vi "TimeStamp To String.vi"(8 "error in (no error)":errorcluster, 11 "Time Stamp":timestamp) -> (0 "error out":errorcluster, 3 "Time string":string)   [LabVIEW 2020, in "Data.lvlib" / "Time Stamp.lvclass"]
doc: "Format a Time Stamp into a String with the format: YYYY-MM-DD hh:mm:ss.ddd"
uses:
  Time Stamp.lvclass
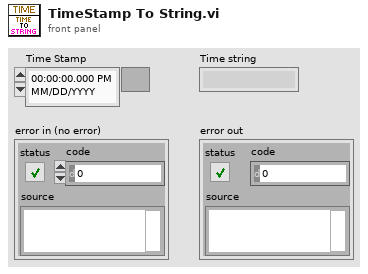
[diagram p1: front panel]
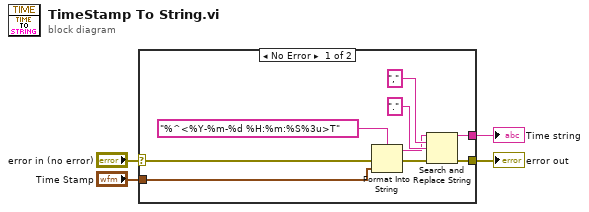
[diagram p0: block diagram]
diagram:
  n1 = case shown="No Error" "error in (no error)" {
    selector: "error in (no error)" -> [w7 w14]
    tunnel: [w13 _] -> w4
    tunnel: [w12 w14] -> w3
    tunnel: "Time Stamp" -> [w5 _]
    frame No Error {
      n2 = Format Into String(format string="%^<%Y-%m-%d %H:%m:%S%3u>T", error in=w7, w5) -> (resulting string=w8:string, error out=w11:errorcluster)  [unwired: 1 in]
      n3 = Search and Replace String(input string=w8, search string=",", replace string="." ("search string"), error in=w11) -> (result string=w13:string, error out=w12:errorcluster)  [unwired: 4 in, 2 out]
    }
    frame Error {
    }
  }
  "Time string" <- w4
  "error out" <- w3
